vi "gSpectrometer.vi"() -> ()   [LabVIEW 2019]
uses:
  Type Definitions.llb/Wavelength Unit.ctt
  Type Definitions.llb/McPherson Grating Density.ctl
  Type Definitions.llb/McPherson Status.ctt
panel:
  in  "McPherson Status":T1
  in  "Current nm":dbl=6000.0 min=0.0 max=26000.0 format="%.2f"
  in  "Current WL":dbl=6000.0 min=0.0 max=26000.0 format="%.2f"
  in  "Current Counter Position":dbl=6000.0 min=0.0 max=26000.0 format="%.2f"
  in  "CurrentStepperPosition":i32 min=-8388607 max=8388607
  in  "Original Counter Position":dbl=6000.0 min=0.0 max=26000.0 format="%.2f"
  in  "Wavelength Unit":T2=enum."nm"
  in  "Grating Density":T3=enum."600"
  in  "McP OK?":bool
  in  "McP Steps/Angstrom":i32=250 min=250 max=250
  in  "McP Port#":refnum<visa-resource-name>="ASRL25::INSTR"
  in  "McP Scan Velocity":i32
  # "Spectrometer Controls"
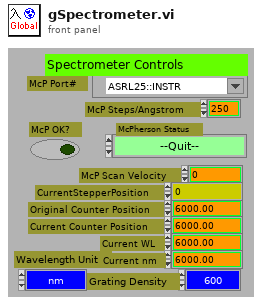
[diagram p1: front panel]
types:
  T1 = typedef "McPherson Status.ctt" = enum8{"--Quit--", "Error", "Initialization", "Standby", "Start Slew", "-Slew", "+Slew", "Slew Done", "Start Scan", "-Slew to Start", "+Slew to Start", "Scanning", "Scan Done", "Scan Pause", "Slew Pause", "Cancel", "Update Z0", "Sleep"}
  T2 = typedef "Wavelength Unit.ctt" = enum8{"Point", "nm", "eV", "meV", "cm_1"}
  T3 = typedef "McPherson Grating Density.ctl" = enum8{"150", "300", "600", "1200", "1800"}
diagram:
